vi "Agilent 546XX Series Acq Dual Wfm Edge Triggered.vi"() -> ()   [LabVIEW 2014]
doc: "DESCRIPTION:\nThis VI shows how to configure the Agilent 546xx Series for a dual-channel waveform acquisition. It uses edge triggering to trigger the acquisition. \n\nINSTRUCTIONS:\n1. Pass a valid VISA session\n2. Enter a vertical offset, range and coupling for the specified channels.\n3. Enter the probe attenuation for the probe attached to the specified channel inputs.\n4. Enter the acquisition start time, desired time per record and the minimum number of points you want in the record.\n5. Enter the trigger level for the edge trigger.\n6. Run the VI.\n7. The acquired waveforms will be displayed in the graph.\n\nNOTES:\nNotice the order of the Agilent 546xx component VIs in the block diagram.\n\nThis VI sets the following controls on the block diagram:\n 20MHz Max Input Frequency.\n 1.0M Ohm Input Impedance.\n 200 ns Trigger Holdoff\n Edge trigger is DC coupled with a positive slope.\nTo change these controls, modify the associated block diagram constants."
uses:
  <instrlib>/Agilent 546XX Series/Agilent 546XX Series.lvlib
panel:
  in  "Serial Configuration":cluster{"Baud Rate":u32, "Flow Control":u16}={"Baud Rate"=0, "Flow Control"=4} {"Flow Control" items=["None", "XON/XOFF", "RTS/CTS", "XON/XOFF & RTS/CTS", "DTR/DSR", "XON/XOFF & DTR/DSR"]; "Baud Rate" items=["9600", "19200", "38400", "57600"]}
  in  "Vertical Offset (0.0 V)":dbl format="%^.3e"
  in  "Vertical Range (2.0 V)":dbl=2.0 format="%^.2e"
  in  "Probe Attenuation (1x)":dbl=1.0 format="%.2f"
  in  "Vertical Offset (0.0 V)":dbl format="%^.3e"
  in  "Vertical Range (2.0 V)":dbl=2.0 format="%^.2e"
  in  "Probe Attenuation (1x)":dbl=1.0 format="%.2f"
  in  "Trigger Level (0.0 V)":dbl format="%^.2e"
  in  "Min Record Length (1000)":i32=1000
  in  "Time Per Record (20.0e-3 s)":dbl=0.02 format="%^.2e"
  in  "Vertical Coupling (DC)":i32(slide)=1
  in  "Vertical Coupling (DC)":i32(slide)=1
  in  "Channel Name (\"CH2\")":string(combo)="CHAN2"
  in  "Channel Name (\"CH1\")":string(combo)="CHAN1"
  out "Waveform Graph":T1(graph)
  in  "VISA Resource Name":refnum<visa-resource-name>
  # "Horizontal Configuration"
  # "Triggering (Channel A)"
  # "Channel A Configuration"
  # "Channel B Configuration"
  # "For instructions,\nselect Show Context Help\nfrom the Help menu."
  # "© 2005, National Instruments, Corporation.  All Rights Reserved."
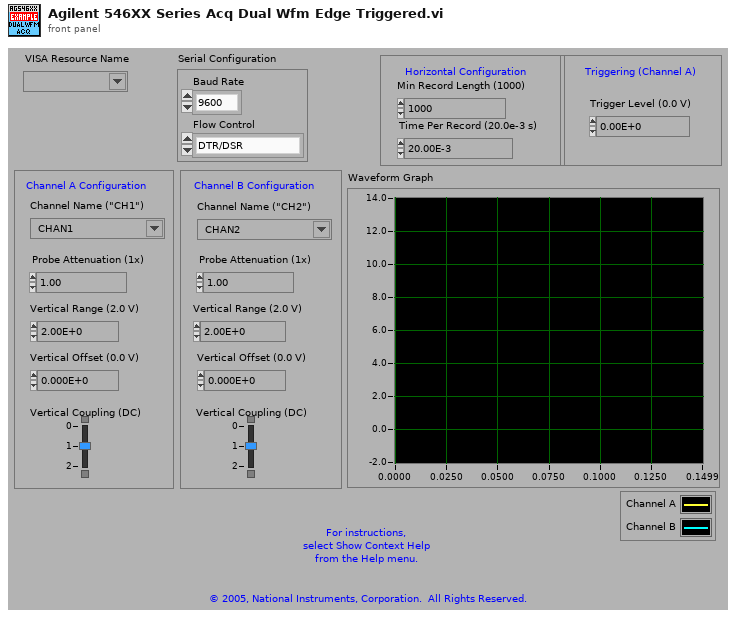
[diagram p1: front panel]
types:
  T1 = cluster{"initial x":dbl, "x increment":dbl, "waveform array":dbl[]}[]
  T2 = cluster{"initial x":dbl, "x increment":dbl, " waveform array  ":dbl[]}
  T3 = cluster{"initial x":dbl, "x increment":dbl, " waveform array  ":dbl[]}[]
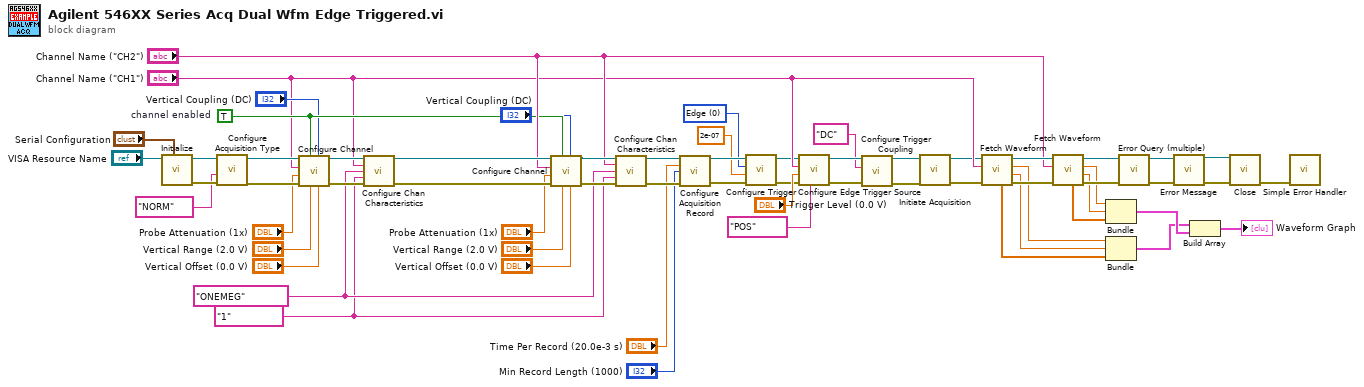
[diagram p0: block diagram]
diagram:
  w13 = 0 items=["Edge", "Glitch", "TV", "AC Line", "Pattern", "Duration", "IIC", "Sequence"] ("Trigger Type (Edge)")
  w48 = "1" ("Max Input Frequency (20.0E+6 Hz)")
  w49 = "ONEMEG" ("Input Impedance (1.0 mega ohm)")
  w37 = TRUE  # channel enabled
  n1 = call <instrlib>:"Initialize.vi"("Serial Configuration"="Serial Configuration", "VISA Resource Name"="VISA Resource Name") -> ("error out"=w63:errorcluster, "VISA Resource Name Out"=w2:refnum<visa-resource-name>)  [unwired: 8 in]
  n2 = call <instrlib>:"Configure Acquisition Type.vi"("error in (no error)"=w63, "Acquisition Type (Sample)"="NORM", "VISA Resource Name"=w2) -> ("error out"=w61:errorcluster, "VISA Resource Name Out"=w59:refnum<visa-resource-name>)  [unwired: 7 in]
  n3 = call <instrlib>:"Configure Channel.vi"("Vertical Offset (0.0 V)"="Vertical Offset (0.0 V)", "Vertical Coupling (DC)"="Vertical Coupling (DC)", "Vertical Range (40 V)"="Vertical Range (2.0 V)", "Channel Enabled (True)"=w37, "error in (no error)"=w61, "Probe Attenuation (1x)"="Probe Attenuation (1x)", "Channel Name (\"Channel 1\")"="Channel Name (\"CH1\")", "VISA Resource Name"=w59) -> ("error out"=w60:errorcluster, "VISA Resource Name Out"=w58:refnum<visa-resource-name>)  [unwired: 2 in]
  n4 = call <instrlib>:"Configure Chan Characteristics.vi"("VISA Resource Name"=w58, "Channel Name (\"Channel 1\")"="Channel Name (\"CH1\")", "Input Impedance (1.0 mega ohm)"=w49, "Max Input Frequency (20.0E+6 Hz)"=w48, "error in (no error)"=w60) -> ("VISA Resource Name Out"=w55:refnum<visa-resource-name>, "error out"=w54:errorcluster)  [unwired: 9 in]
  n5 = call <instrlib>:"Configure Channel.vi"("Vertical Offset (0.0 V)"="Vertical Offset (0.0 V)", "Vertical Coupling (DC)"="Vertical Coupling (DC)", "Vertical Range (40 V)"="Vertical Range (2.0 V)", "Channel Enabled (True)"=w37, "error in (no error)"=w54, "Probe Attenuation (1x)"="Probe Attenuation (1x)", "Channel Name (\"Channel 1\")"="Channel Name (\"CH2\")", "VISA Resource Name"=w55) -> ("error out"=w53:errorcluster, "VISA Resource Name Out"=w52:refnum<visa-resource-name>)  [unwired: 2 in]
  n6 = call <instrlib>:"Configure Chan Characteristics.vi"("VISA Resource Name"=w52, "Channel Name (\"Channel 1\")"="Channel Name (\"CH2\")", "Input Impedance (1.0 mega ohm)"=w49, "Max Input Frequency (20.0E+6 Hz)"=w48, "error in (no error)"=w53) -> ("VISA Resource Name Out"=w51:refnum<visa-resource-name>, "error out"=w50:errorcluster)  [unwired: 9 in]
  n7 = call <instrlib>:"Configure Acquisition Record.vi"("VISA Resource Name"=w51, "Time Per Record (1.0e-3 s)"="Time Per Record (20.0e-3 s)", "Minimum Record Length (2000)"="Min Record Length (1000)", "error in (no error)"=w50) -> ("VISA Resource Name Out"=w14:refnum<visa-resource-name>, "error out"=w15:errorcluster)  [unwired: 10 in]
  n8 = call <instrlib>:"Configure Trigger.vi"("error in (no error)"=w15, "trigger holdoff (60.0E-9 s)"=2e-07, "Trigger Type (Edge)"=w13, "VISA Resource Name"=w14) -> ("error out"=w16:errorcluster, "VISA Resource Name Out"=w17:refnum<visa-resource-name>)  [unwired: 6 in]
  n9 = call <instrlib>:"Configure Edge Trigger Source.vi"("Trigger Slope (Positive)"="POS", "error in (no error)"=w16, "Trigger Level (0.0 V)"="Trigger Level (0.0 V)", "Trigger Source (Channel 1)"="Channel Name (\"CH1\")", "VISA Resource Name"=w17) -> ("error out"=w56:errorcluster, "VISA Resource Name Out"=w57:refnum<visa-resource-name>)  [unwired: 5 in]
  n10 = call <instrlib>:"Configure Trigger Coupling.vi"("error in (no error)"=w56, "Trigger Coupling (DC)"="DC", "VISA Resource Name"=w57) -> ("error out"=w28:errorcluster, "VISA Resource Name Out"=w29:refnum<visa-resource-name>)  [unwired: 7 in]
  n11 = call <instrlib>:"Initiate Acquisition.vi"("error in (no error)"=w28, "VISA Resource Name"=w29) -> ("error out"=w10:errorcluster, "VISA Resource Name Out"=w11:refnum<visa-resource-name>)  [unwired: 8 in]
  n12 = call <instrlib>:"Fetch Waveform.vi"("error in (no error)"=w10, "Channel Name (\"Channel 1\")"="Channel Name (\"CH1\")", "VISA Resource Name"=w11) -> ("error out"=w47:errorcluster, "x increment"=w43:dbl, "initial x"=w44:dbl, "VISA Resource Name Out"=w46:refnum<visa-resource-name>, "waveform array"=w42:dbl[])  [unwired: 3 in, 1 out]
  n13 = call <instrlib>:"Fetch Waveform.vi"("error in (no error)"=w47, "Channel Name (\"Channel 1\")"="Channel Name (\"CH2\")", "VISA Resource Name"=w46) -> ("error out"=w62:errorcluster, "x increment"=w40:dbl, "initial x"=w39:dbl, "VISA Resource Name Out"=w9:refnum<visa-resource-name>, "waveform array"=w41:dbl[])  [unwired: 3 in, 1 out]
  n14 = Bundle("initial x"=w39, "x increment"=w40, "waveform array"=w41) -> (w32:T2)  [unwired: 1 in]
  n15 = Bundle("initial x"=w44, "x increment"=w43, "waveform array"=w42) -> (w31:T2)  [unwired: 1 in]
  n16 = call <instrlib>:"Error Query (multiple).vi"("error in (no error)"=w62, "VISA Resource Name"=w9) -> ("error out"=w6:errorcluster, "VISA Resource Name Out"=w8:refnum<visa-resource-name>)  [unwired: 6 in, 2 out]
  n17 = call <instrlib>:"Error Message.vi"("VISA Resource Name"=w8, "error in (no error)"=w6) -> ("VISA Resource Name Out"=w7:refnum<visa-resource-name>, "error out"=w5:errorcluster)  [unwired: 9 in, 3 out]
  n18 = Build Array(w31, w32) -> (→"Waveform Graph":T3)
  n19 = call <instrlib>:"Close.vi"("error in (no error)"=w5, "VISA Resource Name"=w7) -> ("error out"=w4:errorcluster)  [unwired: 9 in]
  n20 = call <vilib>:"Simple Error Handler.vi"("error in (no error)"=w4) -> ()  [unwired: 4 in, 5 out]
